vi "WriteSubpanels.vi"(8 "error in (no error)":errorcluster, 10 "Subpanels":refnum<class "EmbeddedSMO.lvclass">[](array[class]), 11 "EmbeddedMainUI in":refnum<class "EmbeddedMainUI.lvclass">) -> (0 "error out":errorcluster, 3 "EmbeddedMainUI out":refnum<class "EmbeddedMainUI.lvclass">)   [LabVIEW 2016, in "EmbeddedMainUI.lvclass"]
uses:
  EmbeddedMainUI.lvclass
  <vilib>/Levylab/Embedded SMO UI/EmbeddedSMO.lvclass
  EmbeddedMainUI.lvclass/EmbeddedMainUI.ctl
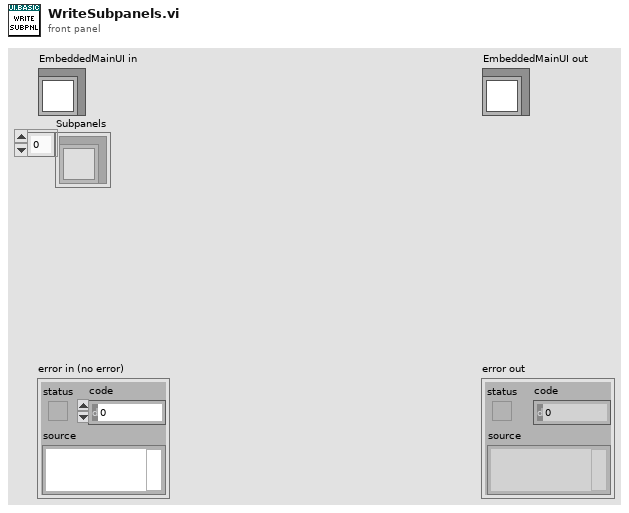
[diagram p1: front panel]
types:
  T1 = typedef "EmbeddedMainUI.lvclass/FrameworkData.ctl" = cluster{"Subpanels":refnum<class "EmbeddedSMO.lvclass">[]}
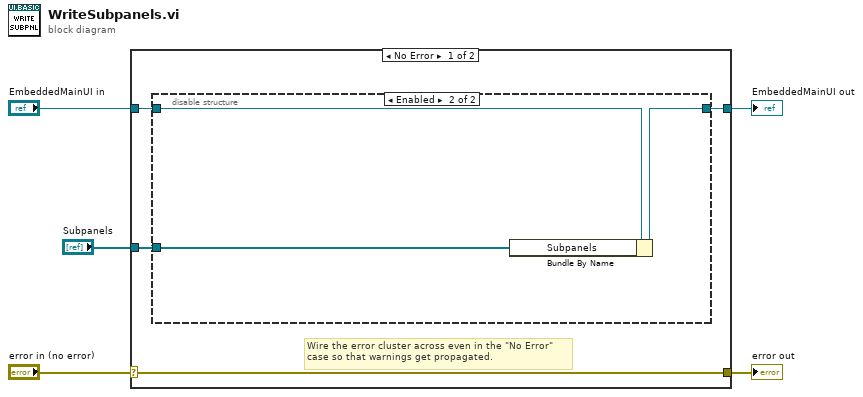
[diagram p0: block diagram]
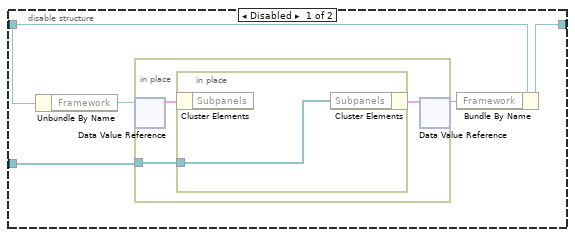
[diagram p2: hidden frame]
diagram:
  n1 = case shown="No Error" "error in (no error)" {
    selector: "error in (no error)" -> [w9 w23]
    tunnel: [w9 w23] -> w4
    tunnel: [w6 w22] -> w2
    tunnel: "EmbeddedMainUI in" -> [w7 w22]
    tunnel: "Subpanels" -> [w8 _]
    frame No Error {
      # "Wire the error cluster across even in the \"No Error\"\ncase so that warnings get propagated."
      n2 = disable-structure shown="Enabled" {
        disable-tunnel: w8 -> [w13 w20]
        disable-tunnel: w7 -> [w12 w21]
        disable-tunnel: [w10 w19] -> w6
        frame Disabled {
          n3 = Unbundle By Name(w12) -> ("Framework"=w14:refnum<data-value>)
          n4 = in-place {
            in-place-border: w13 -> [w17]
            n5 = in-place-dvr #1(w14) -> (w16:T1)  [unwired: 1 out]
            n6 = in-place {
              in-place-border: w17 -> [w18]
              n7 = in-place-cluster #2(w16) -> ()  [unwired: 1 out]
              n8 = in-place-cluster #2("Subpanels"=w18) -> (w15:T1)
            }
            n9 = in-place-dvr #1(w15) -> (w11:refnum<data-value>)  [unwired: 1 out]
          }
          n10 = Bundle By Name(cluster=w12, "Framework"=w11) -> (w10:refnum<class "EmbeddedMainUI.lvclass">)
        }
        frame Enabled {
          n11 = Bundle By Name(cluster=w21, "Subpanels"=w20) -> (w19:refnum<class "EmbeddedMainUI.lvclass">)
        }
      }
    }
    frame Error {
    }
  }
  "error out" <- w4
  "EmbeddedMainUI out" <- w2
